vi "Set Forward Rotation Direction_Multiple.vi"(8 "error in (no error)":errorcluster, 10 "forward rotation directions":T1[](array[typedef]) items=["Clockwise", "Counterclockwise"], 11 "wheels in":refnum<class "NI_Robotics_Wheel.lvclass">[](array[class])) -> (0 "error out":errorcluster, 3 "wheels out":refnum<class "NI_Robotics_Wheel.lvclass">[](array[class]))   [LabVIEW 2017, in "NI_Robotics_Wheel.lvclass"]
uses:
  <vilib>/robotics/Steering/Wheel/NI_Robotics_Wheel.lvclass
  <vilib>/robotics/Steering/Wheel/Rotation Direction.ctl
  <vilib>/robotics/Steering/Wheel/NI_Robotics_Wheel.lvclass/NI_Robotics_Wheel.ctl
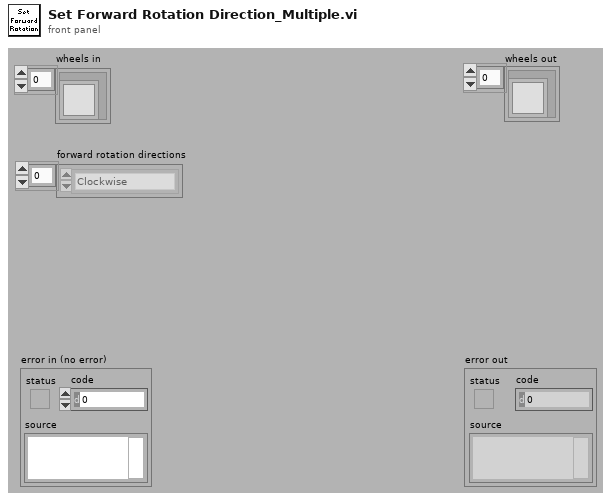
[diagram p1: front panel]
types:
  T1 = typedef "NI_Robotics_Wheel.lvclass/Rotation Direction.ctl" = u16
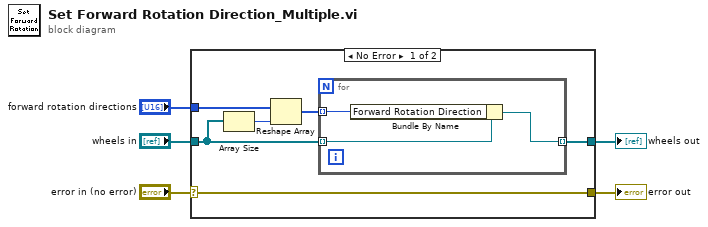
[diagram p0: block diagram]
diagram:
  n1 = case shown="No Error" "error in (no error)" {
    selector: "error in (no error)" -> [w10 w16]
    tunnel: [w10 w16] -> w4
    tunnel: "wheels in" -> [w7 w15]
    tunnel: "forward rotation directions" -> [w9 _]
    tunnel: [w11 w15] -> w1
    frame No Error {
      n2 = Array Size(array=w7) -> (size(s)=w6:i32)
      n3 = Reshape Array(w9, w6) -> (w8:T1[])
      n4 = for {
        tunnel: w7 -> [w14] mode=indexing
        tunnel: w8 -> [w13] mode=indexing
        tunnel: [w12] -> w11 mode=indexing
        n5 = Bundle By Name(cluster=w14, "Forward Rotation Direction"=w13) -> (w12:refnum<class "NI_Robotics_Wheel.lvclass">)
      }
    }
    frame Error {
    }
  }
  "error out" <- w4
  "wheels out" <- w1
